vi "AlazarWriteRegister.vi"(0 "Board Handle":u64, 5 "Offset":u32, 7 "Value":u32, 9 "Password":u32, 11 "error in (no error)":errorcluster) -> (4 "Board Handle Out":u64, 10 "Return Code":u32, 15 "error out":errorcluster)   [LabVIEW 2018]
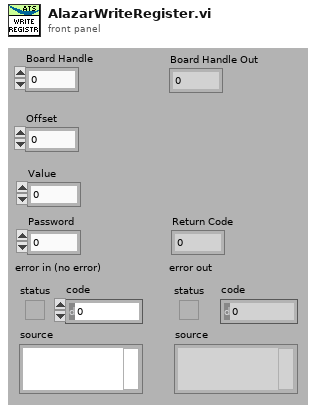
[diagram p1: front panel]
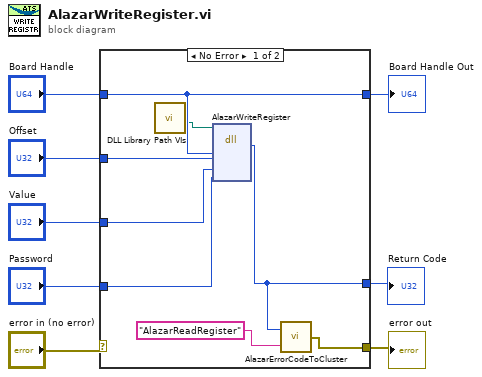
[diagram p0: block diagram]
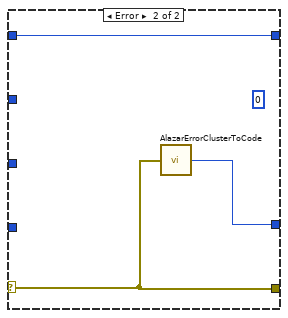
[diagram p2: hidden frame]
diagram:
  n1 = case shown="No Error" "error in (no error)" {
    selector: "error in (no error)" -> [_ w18]
    tunnel: [w11 w18] -> w7
    tunnel: [w16 w19] -> w6
    tunnel: "Board Handle" -> [w16 w19]
    tunnel: [w13 w17] -> w4
    tunnel: "Offset" -> [w15 _]
    tunnel: "Password" -> [w14 _]
    tunnel: "Value" -> [w10 _]
    frame No Error {
      n2 = call "DLL Library Path VIs.vi"() -> ("Alazar"=w9:path)  [unwired: 9 in, 2 out]
      n3 = dll-call lib="C:/Project/SerialSectOCT - FFT GPU/SerialSectOCT/Labview Software/DLL/ATSApi.dll" fn="AlazarWriteRegister"(path in=w9, "handle"=w16, "offset"=w15, "val"=w10, "password"=w14) -> ("return type"=w13:u32)  [unwired: 6 in, 2 out]
      n4 = call "AlazarErrorCodeToCluster.vi"("Message"="AlazarReadRegister", "Error Code"=w13) -> ("error out"=w11:errorcluster)
    }
    frame Error {
      (unwired) u32 0
      n5 = call "AlazarErrorClusterToCode.vi"("error in (no error)"=w18) -> ("Error Code"=w17:u32)
    }
  }
  "Board Handle Out" <- w6
  "error out" <- w7
  "Return Code" <- w4
